vi "RTS Final Station Setups.vi"(0 "Freezer":T4[](array[typedef]) {"Start Time" format="%<%X\n%x>T"; "End Time" format="%<%X\n%x>T"}, 1 "All Door Opener Ctrl in":T1 {"Station 8"."Station Slide"."Chamber 1-1"."Start Time" format="%<%X\n%x>T"; "Station 8"."Station Slide"."Chamber 1-1"."End Time" format="%<%X\n%x>T"; "Station 8"."Station Slide"."Time Count (s)" format="%.2f"; "Station 8"."Station Cab"."Chamber 1-1"."Start Time" format="%<%X\n%x>T"; "Station 8"."Station Cab"."Chamber 1-1"."End Time" format="%<%X\n%x>T"; "Station 8"."Station Cab"."Time Count (s)" format="%.2f"; "Station 8"."Station Freezer"."Chamber 1-1"."Start Time" format="%<%X\n%x>T"; "Station 8"."Station Freezer"."Chamber 1-1"."End Time" format="%<%X\n%x>T"; "Station 8"."Station Freezer"."Time Count (s)" format="%.2f"; "Station 7"."Station Slide"."Chamber 1-1"."Start Time" format="%<%X\n%x>T"; "Station 7"."Station Slide"."Chamber 1-1"."End Time" format="%<%X\n%x>T"; "Station 7"."Station Slide"."Time Count (s)" format="%.2f"; "Station 7"."Station Cab"."Chamber 1-1"."Start Time" format="%<%X\n%x>T"; "Station 7"."Station Cab"."Chamber 1-1"."End Time" format="%<%X\n%x>T"; "Station 7"."Station Cab"."Time Count (s)" format="%.2f"; "Station 7"."Station Freezer"."Chamber 1-1"."Start Time" format="%<%X\n%x>T"; "Station 7"."Station Freezer"."Chamber 1-1"."End Time" format="%<%X\n%x>T"; "Station 7"."Station Freezer"."Time Count (s)" format="%.2f"; "Station 6"."Station Slide"."Chamber 1-1"."Start Time" format="%<%X\n%x>T"; "Station 6"."Station Slide"."Chamber 1-1"."End Time" format="%<%X\n%x>T"; "Station 6"."Station Slide"."Time Count (s)" format="%.2f"; "Station 6"."Station Cab"."Chamber 1-1"."Start Time" format="%<%X\n%x>T"; "Station 6"."Station Cab"."Chamber 1-1"."End Time" format="%<%X\n%x>T"; "Station 6"."Station Cab"."Time Count (s)" format="%.2f"; "Station 6"."Station Freezer"."Chamber 1-1"."Start Time" format="%<%X\n%x>T"; "Station 6"."Station Freezer"."Chamber 1-1"."End Time" format="%<%X\n%x>T"; "Station 6"."Station Freezer"."Time Count (s)" format="%.2f"; "Station 5"."Station Slide"."Chamber 1-1"."Start Time" format="%<%X\n%x>T"; "Station 5"."Station Slide"."Chamber 1-1"."End Time" format="%<%X\n%x>T"; "Station 5"."Station Slide"."Time Count (s)" format="%.2f"; "Station 5"."Station Cab"."Chamber 1-1"."Start Time" format="%<%X\n%x>T"; "Station 5"."Station Cab"."Chamber 1-1"."End Time" format="%<%X\n%x>T"; "Station 5"."Station Cab"."Time Count (s)" format="%.2f"; "Station 5"."Station Freezer"."Chamber 1-1"."Start Time" format="%<%X\n%x>T"; "Station 5"."Station Freezer"."Chamber 1-1"."End Time" format="%<%X\n%x>T"; "Station 5"."Station Freezer"."Time Count (s)" format="%.2f"; "Station 4"."Station Slide"."Chamber 1-1"."Start Time" format="%<%X\n%x>T"; "Station 4"."Station Slide"."Chamber 1-1"."End Time" format="%<%X\n%x>T"; "Station 4"."Station Slide"."Time Count (s)" format="%.2f"; "Station 4"."Station Cab"."Chamber 1-1"."Start Time" format="%<%X\n%x>T"; "Station 4"."Station Cab"."Chamber 1-1"."End Time" format="%<%X\n%x>T"; "Station 4"."Station Cab"."Time Count (s)" format="%.2f"; "Station 4"."Station Freezer"."Chamber 1-1"."Start Time" format="%<%X\n%x>T"; "Station 4"."Station Freezer"."Chamber 1-1"."End Time" format="%<%X\n%x>T"; "Station 4"."Station Freezer"."Time Count (s)" format="%.2f"; "Station 3"."Station Slide"."Chamber 1-1"."Start Time" format="%<%X\n%x>T"; "Station 3"."Station Slide"."Chamber 1-1"."End Time" format="%<%X\n%x>T"; "Station 3"."Station Slide"."Time Count (s)" format="%.2f"; "Station 3"."Station Cab"."Chamber 1-1"."Start Time" format="%<%X\n%x>T"; "Station 3"."Station Cab"."Chamber 1-1"."End Time" format="%<%X\n%x>T"; "Station 3"."Station Cab"."Time Count (s)" format="%.2f"; "Station 3"."Station Freezer"."Chamber 1-1"."Start Time" format="%<%X\n%x>T"; "Station 3"."Station Freezer"."Chamber 1-1"."End Time" format="%<%X\n%x>T"; "Station 3"."Station Freezer"."Time Count (s)" format="%.2f"; "Station 2"."Station Slide"."Chamber 1-1"."Start Time" format="%<%X\n%x>T"; "Station 2"."Station Slide"."Chamber 1-1"."End Time" format="%<%X\n%x>T"; "Station 2"."Station Slide"."Time Count (s)" format="%.2f"; "Station 2"."Station Cab"."Chamber 1-1"."Start Time" format="%<%X\n%x>T"; "Station 2"."Station Cab"."Chamber 1-1"."End Time" format="%<%X\n%x>T"; "Station 2"."Station Cab"."Time Count (s)" format="%.2f"; "Station 2"."Station Freezer"."Chamber 1-1"."Start Time" format="%<%X\n%x>T"; "Station 2"."Station Freezer"."Chamber 1-1"."End Time" format="%<%X\n%x>T"; "Station 2"."Station Freezer"."Time Count (s)" format="%.2f"; "Station 1"."Station Slide"."Chamber 1-1"."Start Time" format="%<%X\n%x>T"; "Station 1"."Station Slide"."Chamber 1-1"."End Time" format="%<%X\n%x>T"; "Station 1"."Station Slide"."Time Count (s)" format="%.2f"; "Station 1"."Station Cab"."Chamber 1-1"."Start Time" format="%<%X\n%x>T"; "Station 1"."Station Cab"."Chamber 1-1"."End Time" format="%<%X\n%x>T"; "Station 1"."Station Cab"."Time Count (s)" format="%.2f"; "Station 1"."Station Freezer"."Chamber 1-1"."Start Time" format="%<%X\n%x>T"; "Station 1"."Station Freezer"."Chamber 1-1"."End Time" format="%<%X\n%x>T"; "Station 1"."Station Freezer"."Time Count (s)" format="%.2f"}, 2 "Station #":u8, 5 "Cab":T4[](array[typedef]) {"Start Time" format="%<%X\n%x>T"; "End Time" format="%<%X\n%x>T"}, 7 "Slide":T4[](array[typedef]) {"Start Time" format="%<%X\n%x>T"; "End Time" format="%<%X\n%x>T"}, 9 "RTS Config Setup Input":T7, 11 "Error In":errorcluster, 12 "Slide Index":i32, 13 "Cab Index":i32, 14 "Freezer Index":i32) -> (3 "All Door Opener Ctrl Out":T1={"Station 1"={"Station Freezer"={"Time Count (s)"=0.0, "Status"="", "Door State"=FALSE, "Delay"=FALSE, "Chamber 1-1"=[], "Index"=0, "Delay Status"=""}, "Station Cab"={"Time Count (s)"=0.0, "Status"="", "Door State"=FALSE, "Delay"=FALSE, "Chamber 1-1"=[], "Index"=0, "Delay Status"=""}, "Station Slide"={"Time Count (s)"=0.0, "Status"="", "Door State"=FALSE, "Delay"=FALSE, "Chamber 1-1"=[], "Index"=0, "Delay Status"=""}, "1st Complete"=FALSE, "2nd Complete"=FALSE, "3rd Complete"=FALSE}, "Station 2"={"Station Freezer"={"Time Count (s)"=0.0, "Status"="", "Door State"=FALSE, "Delay"=FALSE, "Chamber 1-1"=[], "Index"=0, "Delay Status"=""}, "Station Cab"={"Time Count (s)"=0.0, "Status"="", "Door State"=FALSE, "Delay"=FALSE, "Chamber 1-1"=[], "Index"=0, "Delay Status"=""}, "Station Slide"={"Time Count (s)"=0.0, "Status"="", "Door State"=FALSE, "Delay"=FALSE, "Chamber 1-1"=[], "Index"=0, "Delay Status"=""}, "1st Complete"=FALSE, "2nd Complete"=FALSE, "3rd Complete"=FALSE}, "Station 3"={"Station Freezer"={"Time Count (s)"=0.0, "Status"="", "Door State"=FALSE, "Delay"=FALSE, "Chamber 1-1"=[], "Index"=0, "Delay Status"=""}, "Station Cab"={"Time Count (s)"=0.0, "Status"="", "Door State"=FALSE, "Delay"=FALSE, "Chamber 1-1"=[], "Index"=0, "Delay Status"=""}, "Station Slide"={"Time Count (s)"=0.0, "Status"="", "Door State"=FALSE, "Delay"=FALSE, "Chamber 1-1"=[], "Index"=0, "Delay Status"=""}, "1st Complete"=FALSE, "2nd Complete"=FALSE, "3rd Complete"=FALSE}, "Station 4"={"Station Freezer"={"Time Count (s)"=0.0, "Status"="", "Door State"=FALSE, "Delay"=FALSE, "Chamber 1-1"=[], "Index"=0, "Delay Status"=""}, "Station Cab"={"Time Count (s)"=0.0, "Status"="", "Door State"=FALSE, "Delay"=FALSE, "Chamber 1-1"=[], "Index"=0, "Delay Status"=""}, "Station Slide"={"Time Count (s)"=0.0, "Status"="", "Door State"=FALSE, "Delay"=FALSE, "Chamber 1-1"=[], "Index"=0, "Delay Status"=""}, "1st Complete"=FALSE, "2nd Complete"=FALSE, "3rd Complete"=FALSE}, "Station 5"={"Station Freezer"={"Time Count (s)"=0.0, "Status"="", "Door State"=FALSE, "Delay"=TRUE, "Chamber 1-1"=[], "Index"=0, "Delay Status"=""}, "Station Cab"={"Time Count (s)"=0.0, "Status"="", "Door State"=FALSE, "Delay"=TRUE, "Chamber 1-1"=[], "Index"=0, "Delay Status"=""}, "Station Slide"={"Time Count (s)"=0.0, "Status"="", "Door State"=FALSE, "Delay"=TRUE, "Chamber 1-1"=[], "Index"=0, "Delay Status"=""}, "1st Complete"=FALSE, "2nd Complete"=FALSE, "3rd Complete"=FALSE}, "Station 6"={"Station Freezer"={"Time Count (s)"=0.0, "Status"="", "Door State"=FALSE, "Delay"=TRUE, "Chamber 1-1"=[], "Index"=0, "Delay Status"=""}, "Station Cab"={"Time Count (s)"=0.0, "Status"="", "Door State"=FALSE, "Delay"=TRUE, "Chamber 1-1"=[], "Index"=0, "Delay Status"=""}, "Station Slide"={"Time Count (s)"=0.0, "Status"="", "Door State"=FALSE, "Delay"=TRUE, "Chamber 1-1"=[], "Index"=0, "Delay Status"=""}, "1st Complete"=FALSE, "2nd Complete"=FALSE, "3rd Complete"=FALSE}, "Station 7"={"Station Freezer"={"Time Count (s)"=0.0, "Status"="", "Door State"=FALSE, "Delay"=TRUE, "Chamber 1-1"=[], "Index"=0, "Delay Status"=""}, "Station Cab"={"Time Count (s)"=0.0, "Status"="", "Door State"=FALSE, "Delay"=TRUE, "Chamber 1-1"=[], "Index"=0, "Delay Status"=""}, "Station Slide"={"Time Count (s)"=0.0, "Status"="", "Door State"=FALSE, "Delay"=TRUE, "Chamber 1-1"=[], "Index"=0, "Delay Status"=""}, "1st Complete"=FALSE, "2nd Complete"=FALSE, "3rd Complete"=FALSE}, "Station 8"={"Station Freezer"={"Time Count (s)"=0.0, "Status"="", "Door State"=FALSE, "Delay"=TRUE, "Chamber 1-1"=[], "Index"=0, "Delay Status"=""}, "Station Cab"={"Time Count (s)"=0.0, "Status"="", "Door State"=FALSE, "Delay"=TRUE, "Chamber 1-1"=[], "Index"=0, "Delay Status"=""}, "Station Slide"={"Time Count (s)"=0.0, "Status"="", "Door State"=FALSE, "Delay"=TRUE, "Chamber 1-1"=[], "Index"=0, "Delay Status"=""}, "1st Complete"=FALSE, "2nd Complete"=FALSE, "3rd Complete"=FALSE}} {"Station 8"."Station Slide"."Chamber 1-1"."Start Time" format="%<%X\n%x>T"; "Station 8"."Station Slide"."Chamber 1-1"."End Time" format="%<%X\n%x>T"; "Station 8"."Station Slide"."Time Count (s)" format="%.2f"; "Station 8"."Station Cab"."Chamber 1-1"."Start Time" format="%<%X\n%x>T"; "Station 8"."Station Cab"."Chamber 1-1"."End Time" format="%<%X\n%x>T"; "Station 8"."Station Cab"."Time Count (s)" format="%.2f"; "Station 8"."Station Freezer"."Chamber 1-1"."Start Time" format="%<%X\n%x>T"; "Station 8"."Station Freezer"."Chamber 1-1"."End Time" format="%<%X\n%x>T"; "Station 8"."Station Freezer"."Time Count (s)" format="%.2f"; "Station 7"."Station Slide"."Chamber 1-1"."Start Time" format="%<%X\n%x>T"; "Station 7"."Station Slide"."Chamber 1-1"."End Time" format="%<%X\n%x>T"; "Station 7"."Station Slide"."Time Count (s)" format="%.2f"; "Station 7"."Station Cab"."Chamber 1-1"."Start Time" format="%<%X\n%x>T"; "Station 7"."Station Cab"."Chamber 1-1"."End Time" format="%<%X\n%x>T"; "Station 7"."Station Cab"."Time Count (s)" format="%.2f"; "Station 7"."Station Freezer"."Chamber 1-1"."Start Time" format="%<%X\n%x>T"; "Station 7"."Station Freezer"."Chamber 1-1"."End Time" format="%<%X\n%x>T"; "Station 7"."Station Freezer"."Time Count (s)" format="%.2f"; "Station 6"."Station Slide"."Chamber 1-1"."Start Time" format="%<%X\n%x>T"; "Station 6"."Station Slide"."Chamber 1-1"."End Time" format="%<%X\n%x>T"; "Station 6"."Station Slide"."Time Count (s)" format="%.2f"; "Station 6"."Station Cab"."Chamber 1-1"."Start Time" format="%<%X\n%x>T"; "Station 6"."Station Cab"."Chamber 1-1"."End Time" format="%<%X\n%x>T"; "Station 6"."Station Cab"."Time Count (s)" format="%.2f"; "Station 6"."Station Freezer"."Chamber 1-1"."Start Time" format="%<%X\n%x>T"; "Station 6"."Station Freezer"."Chamber 1-1"."End Time" format="%<%X\n%x>T"; "Station 6"."Station Freezer"."Time Count (s)" format="%.2f"; "Station 5"."Station Slide"."Chamber 1-1"."Start Time" format="%<%X\n%x>T"; "Station 5"."Station Slide"."Chamber 1-1"."End Time" format="%<%X\n%x>T"; "Station 5"."Station Slide"."Time Count (s)" format="%.2f"; "Station 5"."Station Cab"."Chamber 1-1"."Start Time" format="%<%X\n%x>T"; "Station 5"."Station Cab"."Chamber 1-1"."End Time" format="%<%X\n%x>T"; "Station 5"."Station Cab"."Time Count (s)" format="%.2f"; "Station 5"."Station Freezer"."Chamber 1-1"."Start Time" format="%<%X\n%x>T"; "Station 5"."Station Freezer"."Chamber 1-1"."End Time" format="%<%X\n%x>T"; "Station 5"."Station Freezer"."Time Count (s)" format="%.2f"; "Station 4"."Station Slide"."Chamber 1-1"."Start Time" format="%<%X\n%x>T"; "Station 4"."Station Slide"."Chamber 1-1"."End Time" format="%<%X\n%x>T"; "Station 4"."Station Slide"."Time Count (s)" format="%.2f"; "Station 4"."Station Cab"."Chamber 1-1"."Start Time" format="%<%X\n%x>T"; "Station 4"."Station Cab"."Chamber 1-1"."End Time" format="%<%X\n%x>T"; "Station 4"."Station Cab"."Time Count (s)" format="%.2f"; "Station 4"."Station Freezer"."Chamber 1-1"."Start Time" format="%<%X\n%x>T"; "Station 4"."Station Freezer"."Chamber 1-1"."End Time" format="%<%X\n%x>T"; "Station 4"."Station Freezer"."Time Count (s)" format="%.2f"; "Station 3"."Station Slide"."Chamber 1-1"."Start Time" format="%<%X\n%x>T"; "Station 3"."Station Slide"."Chamber 1-1"."End Time" format="%<%X\n%x>T"; "Station 3"."Station Slide"."Time Count (s)" format="%.2f"; "Station 3"."Station Cab"."Chamber 1-1"."Start Time" format="%<%X\n%x>T"; "Station 3"."Station Cab"."Chamber 1-1"."End Time" format="%<%X\n%x>T"; "Station 3"."Station Cab"."Time Count (s)" format="%.2f"; "Station 3"."Station Freezer"."Chamber 1-1"."Start Time" format="%<%X\n%x>T"; "Station 3"."Station Freezer"."Chamber 1-1"."End Time" format="%<%X\n%x>T"; "Station 3"."Station Freezer"."Time Count (s)" format="%.2f"; "Station 2"."Station Slide"."Chamber 1-1"."Start Time" format="%<%X\n%x>T"; "Station 2"."Station Slide"."Chamber 1-1"."End Time" format="%<%X\n%x>T"; "Station 2"."Station Slide"."Time Count (s)" format="%.2f"; "Station 2"."Station Cab"."Chamber 1-1"."Start Time" format="%<%X\n%x>T"; "Station 2"."Station Cab"."Chamber 1-1"."End Time" format="%<%X\n%x>T"; "Station 2"."Station Cab"."Time Count (s)" format="%.2f"; "Station 2"."Station Freezer"."Chamber 1-1"."Start Time" format="%<%X\n%x>T"; "Station 2"."Station Freezer"."Chamber 1-1"."End Time" format="%<%X\n%x>T"; "Station 2"."Station Freezer"."Time Count (s)" format="%.2f"; "Station 1"."Station Slide"."Chamber 1-1"."Start Time" format="%<%X\n%x>T"; "Station 1"."Station Slide"."Chamber 1-1"."End Time" format="%<%X\n%x>T"; "Station 1"."Station Slide"."Time Count (s)" format="%.2f"; "Station 1"."Station Cab"."Chamber 1-1"."Start Time" format="%<%X\n%x>T"; "Station 1"."Station Cab"."Chamber 1-1"."End Time" format="%<%X\n%x>T"; "Station 1"."Station Cab"."Time Count (s)" format="%.2f"; "Station 1"."Station Freezer"."Chamber 1-1"."Start Time" format="%<%X\n%x>T"; "Station 1"."Station Freezer"."Chamber 1-1"."End Time" format="%<%X\n%x>T"; "Station 1"."Station Freezer"."Time Count (s)" format="%.2f"}, 4 "States":string, 10 "RTS Config Setup Output":T7, 15 "Error Out":errorcluster)   [LabVIEW 2016]
uses:
  Type Definitions/RTS All Station Door Opener Ctrl.ctl
  Type Definitions/RTS Station Relay Ops.ctl
  Type Definitions/RTS Door Opener Indicator.ctl
  Type Definitions/RTS Door Ops Client.ctl
  Type Definitions/RTS Door Opening Schedule.ctl
  Type Definitions/RTS Door Ops Sequence.ctl
  Type Definitions/RTS Configuration Setup.ctl
  Type Definitions/RTS Wago Config.ctl
  Type Definitions/RTS APLUS Config.ctl
  Type Definitions/RTS Yokogawa MX Config.ctl
  Type Definitions/RTS Replay Server Control.ctl
  Type Definitions/RTS Server Configuration.ctl
  Type Definitions/RTS Station Settions TCP Comms.ctl
  Type Definitions/RTS Chamber Save Status.ctl
  Type Definitions/RTS Test Pattern.ctl
panel:
  # "Chamber Conditions:"
  # "Chamber Conditions:"
  # "Chamber Conditions:"
  # "Chamber Conditions:"
  # "Chamber Conditions:"
  # "Chamber Conditions:"
  # "Chamber Conditions:"
  # "Chamber Conditions:"
  # "Chamber Conditions:"
  # "Chamber Conditions:"
  # "Chamber Conditions:"
  # "Chamber Conditions:"
  # "Chamber Conditions:"
  # "Chamber Conditions:"
  # "Chamber Conditions:"
  # "Chamber Conditions:"
  # "Chamber Conditions:"
  # "Chamber Conditions:"
  # "Chamber Conditions:"
  # "Chamber Conditions:"
  # "Chamber Conditions:"
  # "Chamber Conditions:"
  # "Chamber Conditions:"
  # "Chamber Conditions:"
  # "Chamber Conditions:"
  # "Chamber Conditions:"
  # "Chamber Conditions:"
  # "Chamber Conditions:"
  # "Chamber Conditions:"
  # "Chamber Conditions:"
  # "Chamber Conditions:"
  # "Chamber Conditions:"
  # "Chamber Conditions:"
  # "Chamber Conditions:"
  # "Chamber Conditions:"
  # "Chamber Conditions:"
  # "Chamber Conditions:"
  # "Chamber Conditions:"
  # "Chamber Conditions:"
  # "Chamber Conditions:"
  # "Chamber Conditions:"
  # "Chamber Conditions:"
  # "Chamber Conditions:"
  # "Chamber Conditions:"
  # "Chamber Conditions:"
  # "Chamber Conditions:"
  # "Chamber Conditions:"
  # "Chamber Conditions:"
  # "Chamber Conditions:"
  # "Chamber Conditions:"
  # "Chamber Conditions:"
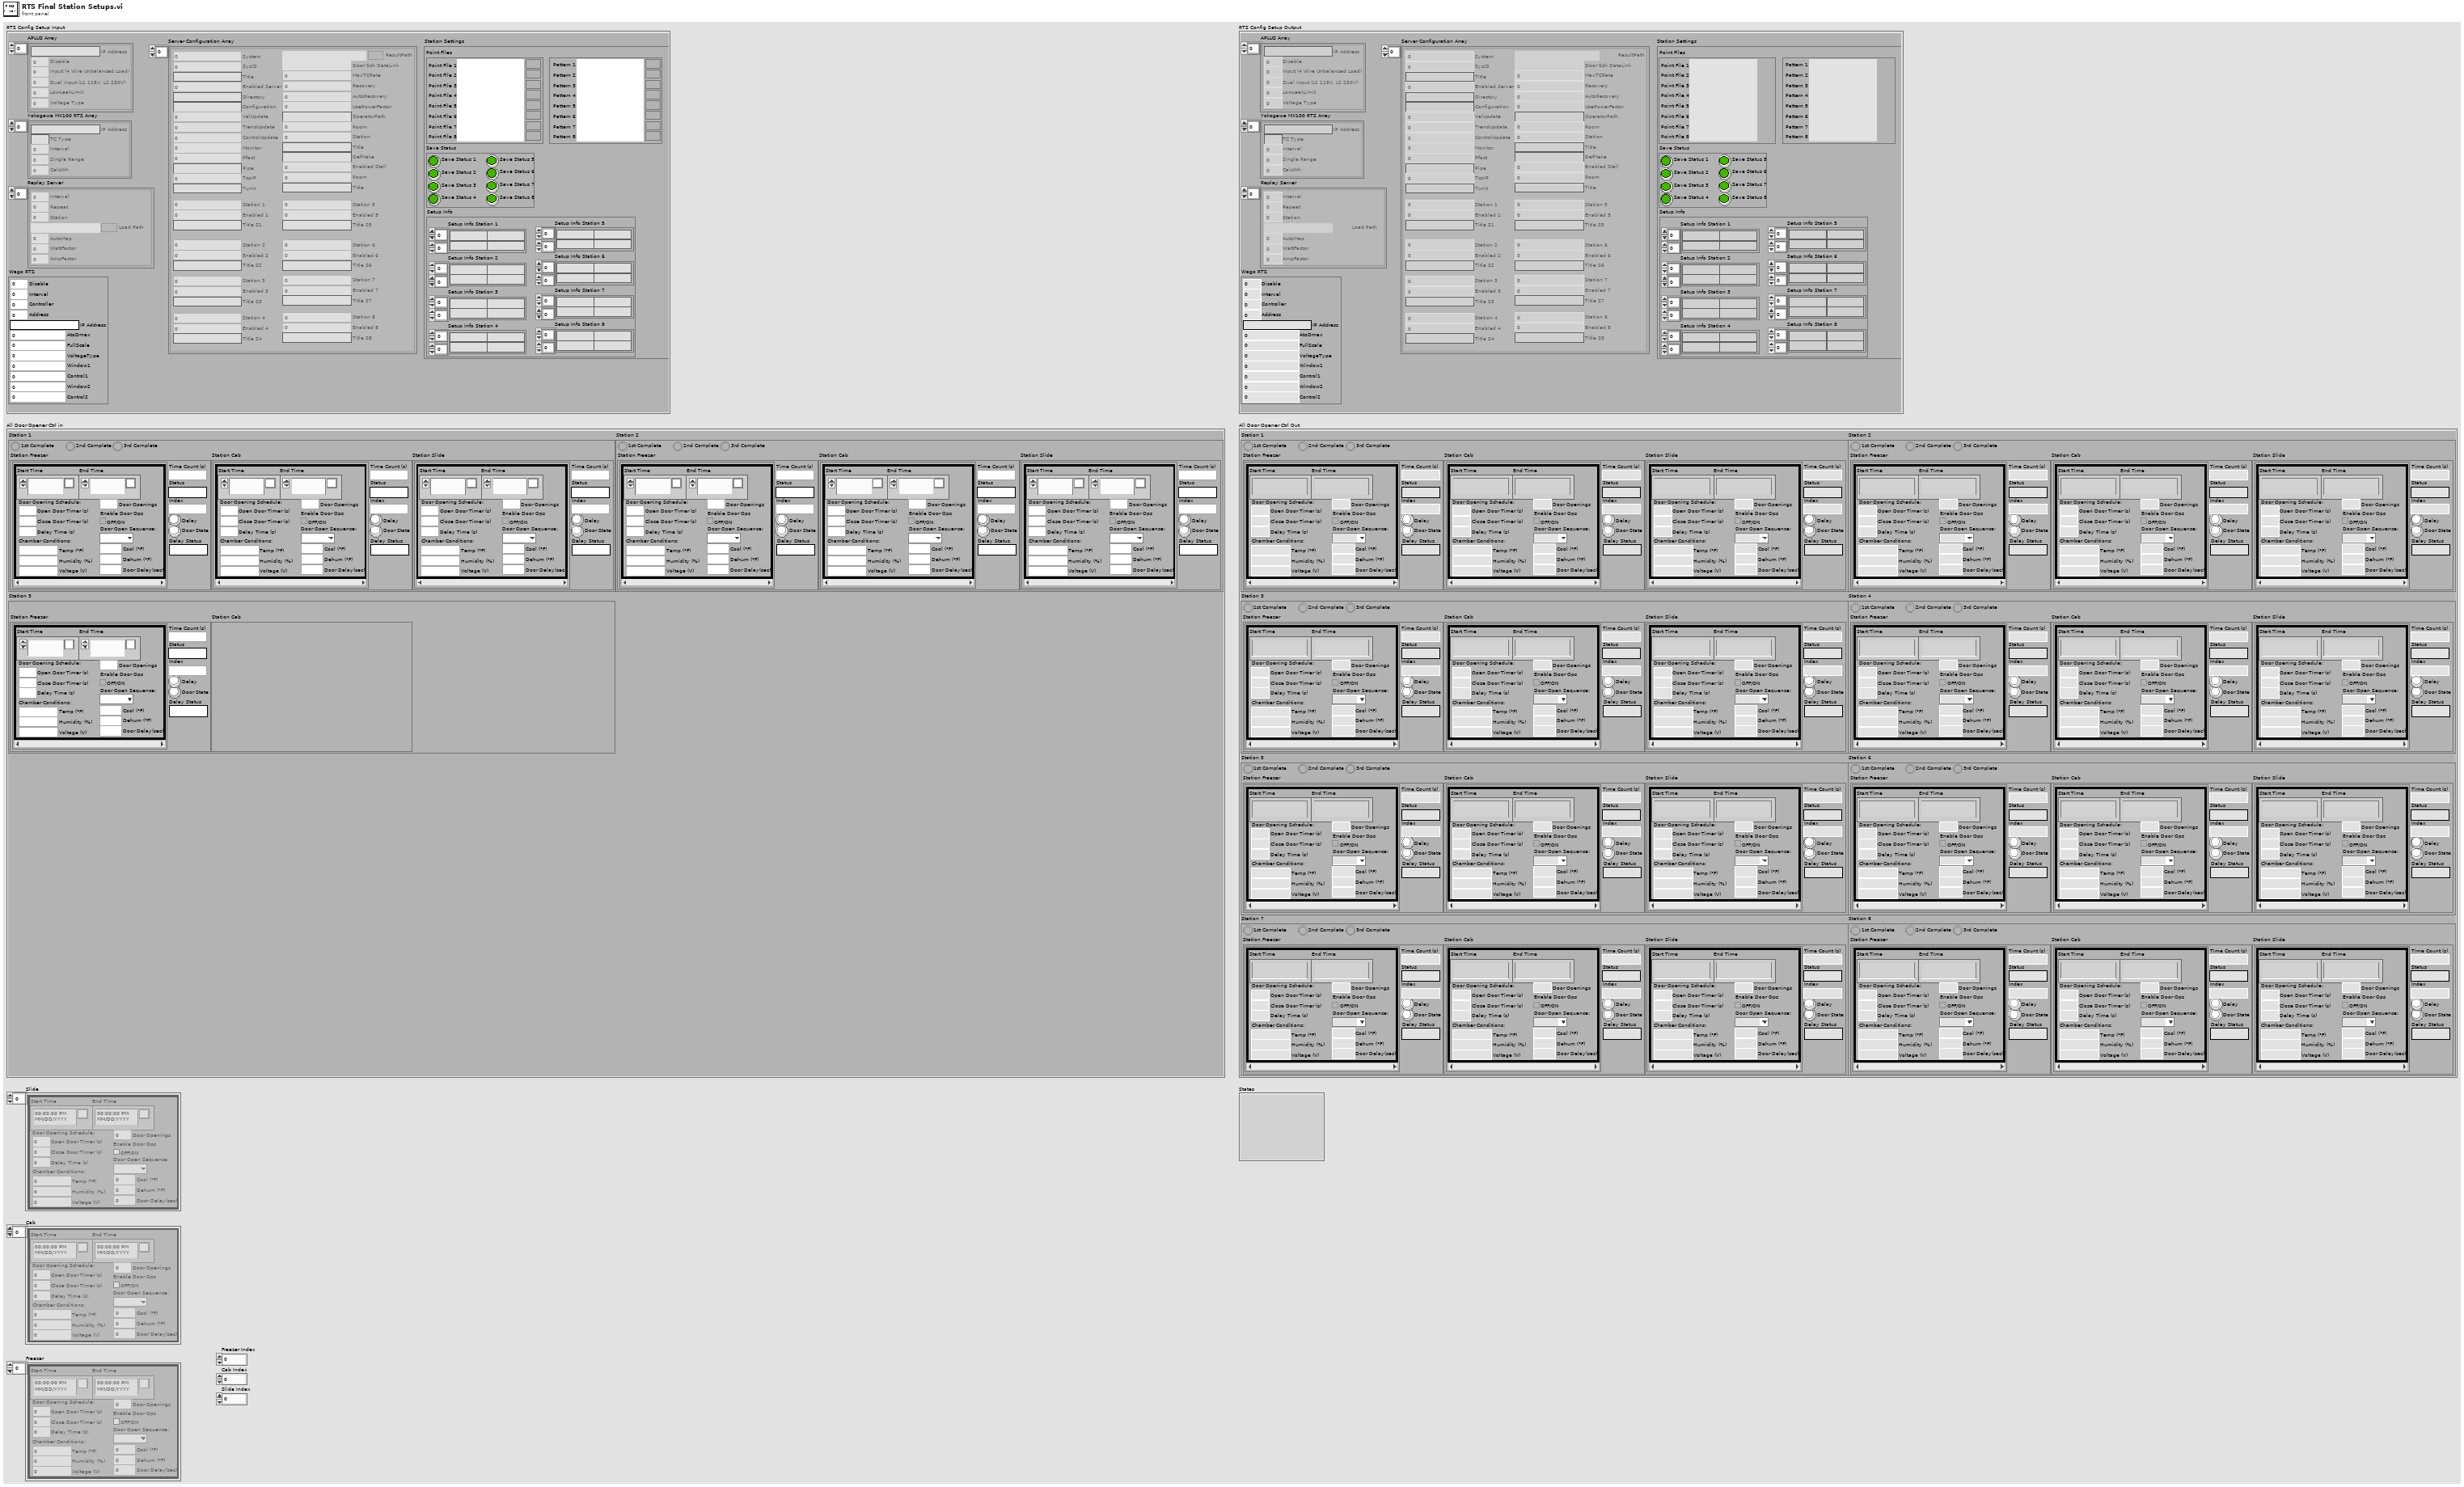
[diagram p1: front panel]
types:
  T1 = typedef "RTS All Station Door Opener Ctrl.ctl" = cluster{"Station 1":T2, "Station 2":T2, "Station 3":T2, "Station 4":T2, "Station 5":T2, "Station 6":T2, "Station 7":T2, "Station 8":T2}
  T2 = typedef "RTS Station Relay Ops.ctl" = cluster{"Station Freezer":T3, "Station Cab":T3, "Station Slide":T3, "1st Complete":bool, "2nd Complete":bool, "3rd Complete":bool}
  T3 = typedef "RTS Door Opener Indicator.ctl" = cluster{"Time Count (s)":dbl, "Status":string, "Door State":bool, "Delay":bool, "Chamber 1-1":T4[], "Index":i32, "Delay Status":string}
  T4 = typedef "RTS Door Ops Client.ctl" = cluster{"End Time":timestamp, "Start Time":timestamp, "Door Opening Schedule:":T5, "Enable Door Ops":bool, "Door Openings":u32, "Temp (°F)":dbl, "Humidity (%)":dbl, "Voltage (V)":dbl, "Door Open Sequence:":T6, "Door Delay(sec)":dbl, "Dehum (°F)":dbl, "Cool (°F)":dbl}
  T5 = typedef "RTS Door Opening Schedule.ctl" = cluster{"Open Door Timer (s)":dbl, "Delay Time (s)":dbl, "Close Door Timer (s)":dbl}
  T6 = typedef "RTS Door Ops Sequence.ctl" = enum16{"", "1st", "2nd", "3rd"}
  T7 = typedef "RTS Configuration Setup.ctl" = cluster{"Wago RTS":T8, "APLUS Array":T9[], "Yokogawa MX100 RTS Array":T10[], "Replay Server":T11[], "Server Configuration Array":T12[], "Station Settings":T13}
  T8 = typedef "RTS Wago Config.ctl" = cluster{"Disable":u16, "Interval":u16, "Controller":u16, "Address":u16, "IP Address":string, "AtoDmax":u16, "FullScale":u16, "VoltageType":u16, "Window1":u16, "Control1":u16, "Window2":u16, "Control2":u16}
  T9 = typedef "RTS APLUS Config.ctl" = cluster{"Disable":u16, "IP Address":string, "Input (4 Wire Unbalanced Load)":u16, "Dual Input (L1 115V, L2 230V)":u16, "LowLeakLimit":dbl, "Voltage Type":u16}
  T10 = typedef "RTS Yokogawa MX Config.ctl" = cluster{"IP Address":string, "TC Type":string, "Interval":u16, "Single Range":u16, "CalcWh":u16}
  T11 = typedef "RTS Replay Server Control.ctl" = cluster{"Interval":i16, "Repeat":u16, "Station":u16, "Load Path":path, "AutoMap":u16, "WattFactor":dbl, "AmpFactor":dbl}
  T12 = typedef "RTS Server Configuration.ctl" = cluster{"System":u16, "SysID":u16, "Title":string, "Enabled Server":u16, "Directory":string, "Configuration":string, "ValUpdate":u16, "TrendUpdate":u16, "ControlUpdate":u16, "Monitor":u16, "Pfact":u16, "Pipe":string, "TcpIP":u16, "Tunit":string, "ResultPath":path, "Door Sch DataLink":path, "MaxTCRate":u16, "Recovery":u16, "AutoRecovery":u16, "UsePowerFactor":u16, "OperatorPath":string, "Room":u16, "Station":u16, "Title":string, "DefMake":string, "Enabled Stall":u16, "Room":u16, "Title":string, "Station 1":u16, "Enabled 1":u16, "Station 2":u16, "Enabled 2":u16, "Station 3":u16, "Enabled 3":u16, "Station 4":u16, "Enabled 4":u16, "Station 5":u16, "Enabled 5":u16, "Station 6":u16, "Enabled 6":u16, "Station 7":u16, "Enabled 7":u16, "Station 8":u16, "Enabled 8":u16, "Title S1":string, "Title S2":string, "Title S3":string, "Title S5":string, "Title S6":string, "Title S7":string, "Title S8":string, "Title S4":string}
  T13 = typedef "RTS Station Settions TCP Comms.ctl" = cluster{"Point Files":cluster{"Point File 1":path, "Point File 2":path, "Point File 3":path, "Point File 4":path, "Point File 5":path, "Point File 6":path, "Point File 7":path, "Point File 8":path}, "Save Status":T14, "Setup Info":cluster{"Setup Info Station 1":string[][], "Setup Info Station 2":string[][], "Setup Info Station 3":string[][], "Setup Info Station 4":string[][], "Setup Info Station 5":string[][], "Setup Info Station 6":string[][], "Setup Info Station 7":string[][], "Setup Info Station 8":string[][]}, "Chamber Test Pattern":T15}
  T14 = typedef "RTS Chamber Save Status.ctl" = cluster{"Save Status 1":bool, "Save Status 2":bool, "Save Status 3":bool, "Save Status 4":bool, "Save Status 5":bool, "Save Status 6":bool, "Save Status 7":bool, "Save Status 8":bool}
  T15 = typedef "RTS Test Pattern.ctl" = cluster{" Pattern 1":path, "Pattern 2":path, "Pattern 3":path, "Pattern 4":path, "Pattern 5":path, "Pattern 6":path, "Pattern 7":path, "Pattern 8":path}
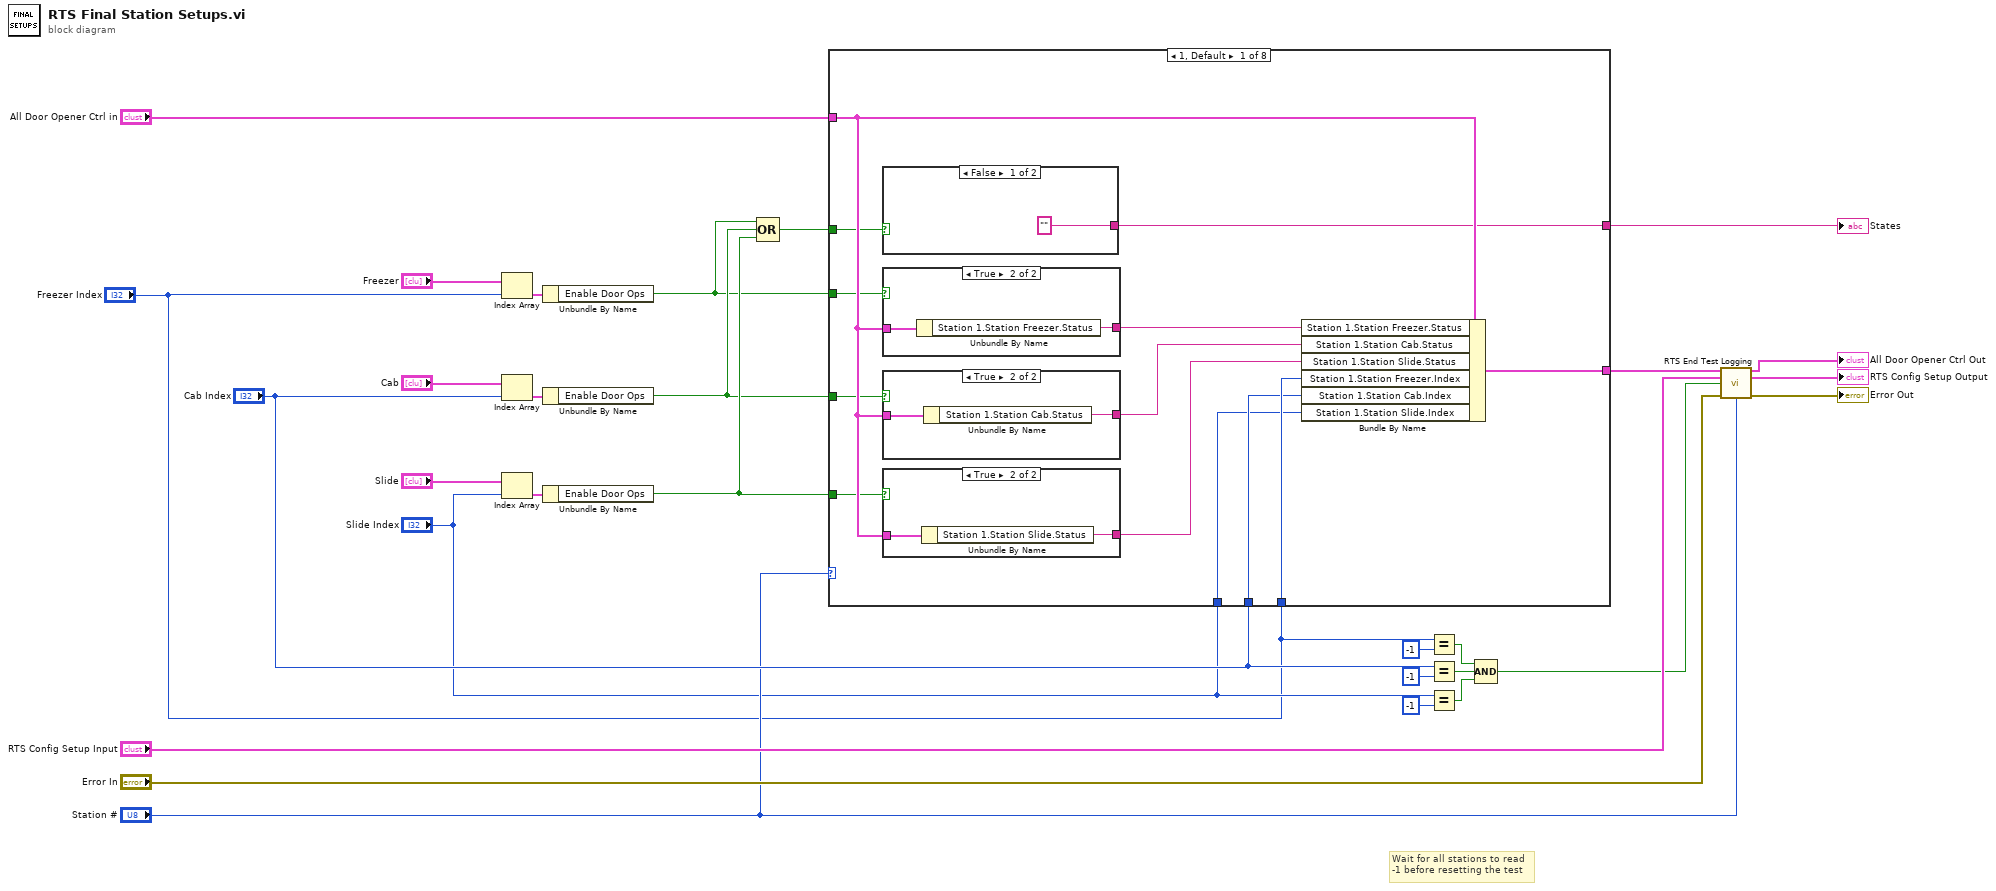
[diagram p0: block diagram]
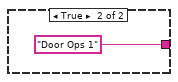
[diagram p2: hidden frame]
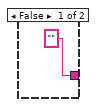
[diagram p3: hidden frame]
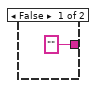
[diagram p4: hidden frame]
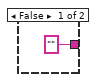
[diagram p5: hidden frame]
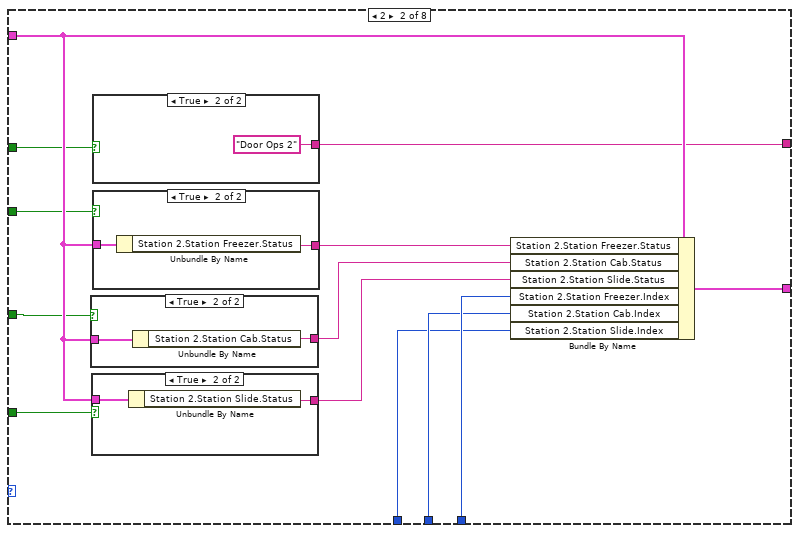
[diagram p6: hidden frame]
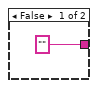
[diagram p7: hidden frame]
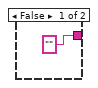
[diagram p8: hidden frame]
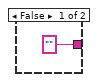
[diagram p9: hidden frame]
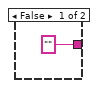
[diagram p10: hidden frame]
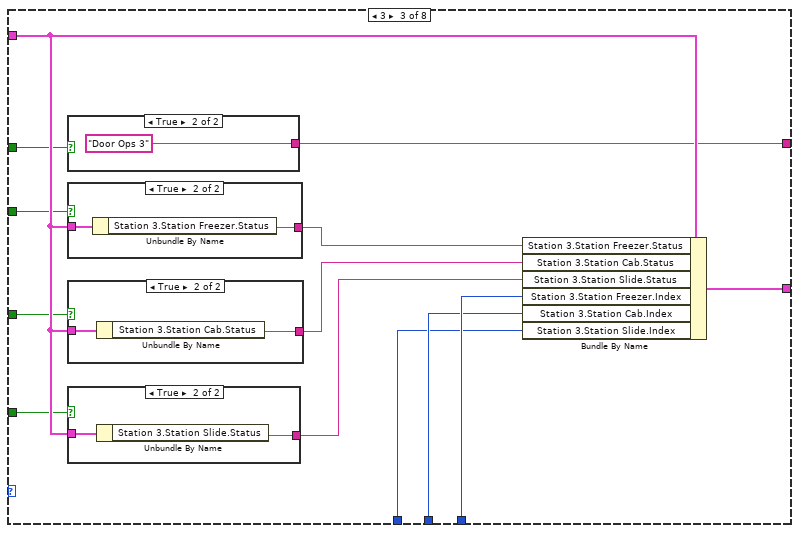
[diagram p11: hidden frame]
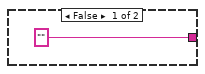
[diagram p12: hidden frame]
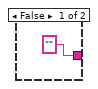
[diagram p13: hidden frame]
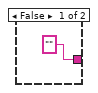
[diagram p14: hidden frame]
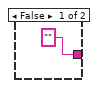
[diagram p15: hidden frame]
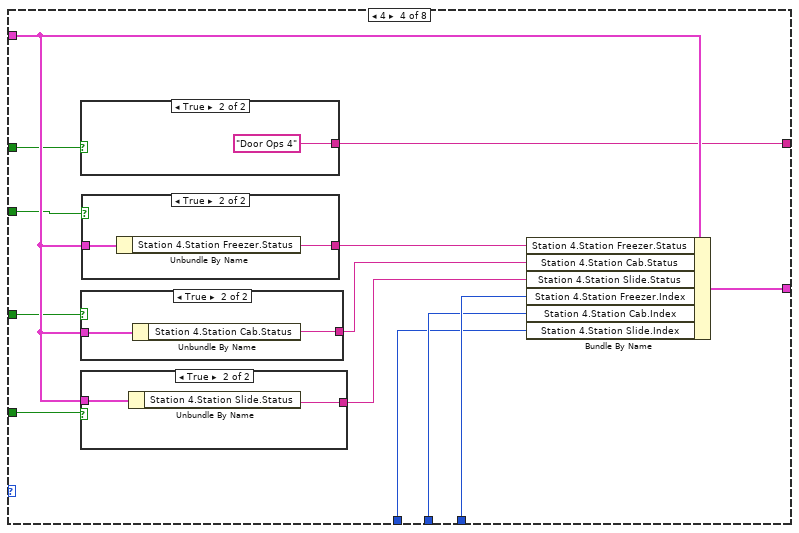
[diagram p16: hidden frame]
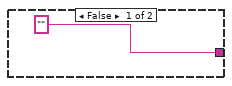
[diagram p17: hidden frame]
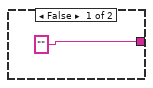
[diagram p18: hidden frame]
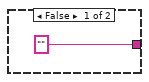
[diagram p19: hidden frame]
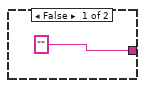
[diagram p20: hidden frame]
diagram:
  # "Wait for all stations to read\n-1 before resetting the test"
  n1 = Index Array(array="Freezer", index="Freezer Index") -> (element=w19:T4)
  n2 = Index Array(array="Cab", index="Cab Index") -> (element=w21:T4)
  n3 = Index Array(array="Slide", index="Slide Index") -> (element=w20:T4)
  n4 = Unbundle By Name(w19) -> ("Enable Door Ops"=w22:bool)
  n5 = Unbundle By Name(w21) -> ("Enable Door Ops"=w23:bool)
  n6 = Unbundle By Name(w20) -> ("Enable Door Ops"=w24:bool)
  n7 = Compound Arithmetic op=OR(w22, w23, w24) -> (w17:bool)
  n8 = case shown="1, Default" "Station #" {
    tunnel: "All Door Opener Ctrl in" -> [w39 w63 w87 w110 w134 w158 w183 w207]
    tunnel: w24 -> [w38 w55 w86 w106 w133 w157 w179 w203]
    tunnel: w23 -> [w37 w56 w85 w107 w132 w156 w178 w202]
    tunnel: w22 -> [w36 w57 w84 w108 w131 w155 w177 w201]
    tunnel: [w35 w62 w81 w105 w129 w154 w180 w205] -> w18
    tunnel: w17 -> [w34 w54 w83 w109 w130 w153 w181 w204]
    tunnel: "Freezer Index" -> [w33 w60 w80 w104 w128 w152 w176 w200]
    tunnel: "Cab Index" -> [w32 w59 w79 w103 w127 w151 w175 w199]
    tunnel: "Slide Index" -> [w31 w58 w78 w102 w126 w150 w174 w198]
    tunnel: [w30 w61 w82 w111 w135 w159 w182 w206] -> w5
    frame 1, Default {
      n9 = case shown="False" w34 {
        tunnel: ["" ("State(s) in Front (\"\")") "Door Ops 1" ("State(s) in Front (\"\")")] -> w35
        frame False {
        }
        frame True {
        }
      }
      n10 = case shown="True" w36 {
        tunnel: ["" w52] -> w40
        tunnel: w39 -> [_ w53]
        frame False {
        }
        frame True {
          n11 = Unbundle By Name(w53) -> ("Station 1.Station Freezer.Status"=w52:string)
        }
      }
      n12 = case shown="True" w37 {
        tunnel: ["" w49] -> w41
        tunnel: w39 -> [_ w50]
        frame False {
        }
        frame True {
          n13 = Unbundle By Name(w50) -> ("Station 1.Station Cab.Status"=w49:string)
        }
      }
      n14 = case shown="True" w38 {
        tunnel: ["" w46] -> w42
        tunnel: w39 -> [_ w47]
        frame False {
        }
        frame True {
          n15 = Unbundle By Name(w47) -> ("Station 1.Station Slide.Status"=w46:string)
        }
      }
      n16 = Bundle By Name(cluster=w39, "Station 1.Station Freezer.Status"=w40, "Station 1.Station Cab.Status"=w41, "Station 1.Station Slide.Status"=w42, "Station 1.Station Freezer.Index"=w33, "Station 1.Station Cab.Index"=w32, "Station 1.Station Slide.Index"=w31) -> (w30:T1)
    }
    frame 2 {
      n17 = case shown="True" w56 {
        tunnel: ["" w73] -> w65
        tunnel: w63 -> [_ w74]
        frame False {
        }
        frame True {
          n18 = Unbundle By Name(w74) -> ("Station 2.Station Cab.Status"=w73:string)
        }
      }
      n19 = case shown="True" w55 {
        tunnel: ["" w70] -> w66
        tunnel: w63 -> [_ w71]
        frame False {
        }
        frame True {
          n20 = Unbundle By Name(w71) -> ("Station 2.Station Slide.Status"=w70:string)
        }
      }
      n21 = case shown="True" w54 {
        tunnel: ["" ("State(s) in Front (\"\")") "Door Ops 2" ("State(s) in Front (\"\")")] -> w62
        frame False {
        }
        frame True {
        }
      }
      n22 = case shown="True" w57 {
        tunnel: ["" w76] -> w64
        tunnel: w63 -> [_ w77]
        frame False {
        }
        frame True {
          n23 = Unbundle By Name(w77) -> ("Station 2.Station Freezer.Status"=w76:string)
        }
      }
      n24 = Bundle By Name(cluster=w63, "Station 2.Station Freezer.Status"=w64, "Station 2.Station Cab.Status"=w65, "Station 2.Station Slide.Status"=w66, "Station 2.Station Freezer.Index"=w60, "Station 2.Station Cab.Index"=w59, "Station 2.Station Slide.Index"=w58) -> (w61:T1)
    }
    frame 3 {
      n25 = case shown="True" w83 {
        tunnel: ["" ("State(s) in Front (\"\")") "Door Ops 3" ("State(s) in Front (\"\")")] -> w81
        frame False {
        }
        frame True {
        }
      }
      n26 = case shown="True" w84 {
        tunnel: ["" w100] -> w88
        tunnel: w87 -> [_ w101]
        frame False {
        }
        frame True {
          n27 = Unbundle By Name(w101) -> ("Station 3.Station Freezer.Status"=w100:string)
        }
      }
      n28 = case shown="True" w85 {
        tunnel: ["" w97] -> w89
        tunnel: w87 -> [_ w98]
        frame False {
        }
        frame True {
          n29 = Unbundle By Name(w98) -> ("Station 3.Station Cab.Status"=w97:string)
        }
      }
      n30 = case shown="True" w86 {
        tunnel: ["" w94] -> w90
        tunnel: w87 -> [_ w95]
        frame False {
        }
        frame True {
          n31 = Unbundle By Name(w95) -> ("Station 3.Station Slide.Status"=w94:string)
        }
      }
      n32 = Bundle By Name(cluster=w87, "Station 3.Station Freezer.Status"=w88, "Station 3.Station Cab.Status"=w89, "Station 3.Station Slide.Status"=w90, "Station 3.Station Freezer.Index"=w80, "Station 3.Station Cab.Index"=w79, "Station 3.Station Slide.Index"=w78) -> (w82:T1)
    }
    frame 4 {
      n33 = case shown="True" w109 {
        tunnel: ["" ("State(s) in Front (\"\")") "Door Ops 4" ("State(s) in Front (\"\")")] -> w105
        frame False {
        }
        frame True {
        }
      }
      n34 = case shown="True" w107 {
        tunnel: ["" w121] -> w113
        tunnel: w110 -> [_ w122]
        frame False {
        }
        frame True {
          n35 = Unbundle By Name(w122) -> ("Station 4.Station Cab.Status"=w121:string)
        }
      }
      n36 = case shown="True" w106 {
        tunnel: ["" w118] -> w112
        tunnel: w110 -> [_ w119]
        frame False {
        }
        frame True {
          n37 = Unbundle By Name(w119) -> ("Station 4.Station Slide.Status"=w118:string)
        }
      }
      n38 = case shown="True" w108 {
        tunnel: ["" w124] -> w114
        tunnel: w110 -> [_ w125]
        frame False {
        }
        frame True {
          n39 = Unbundle By Name(w125) -> ("Station 4.Station Freezer.Status"=w124:string)
        }
      }
      n40 = Bundle By Name(cluster=w110, "Station 4.Station Freezer.Status"=w114, "Station 4.Station Cab.Status"=w113, "Station 4.Station Slide.Status"=w112, "Station 4.Station Freezer.Index"=w104, "Station 4.Station Cab.Index"=w103, "Station 4.Station Slide.Index"=w102) -> (w111:T1)
    }
    frame 5 {
      n41 = case shown="True" w132 {
        tunnel: ["" w145] -> w137
        tunnel: w134 -> [_ w146]
        frame False {
        }
        frame True {
          n42 = Unbundle By Name(w146) -> ("Station 5.Station Cab.Status"=w145:string)
        }
      }
      n43 = case shown="True" w133 {
        tunnel: ["" w142] -> w136
        tunnel: w134 -> [_ w143]
        frame False {
        }
        frame True {
          n44 = Unbundle By Name(w143) -> ("Station 5.Station Slide.Status"=w142:string)
        }
      }
      n45 = case shown="False" w130 {
        tunnel: ["" ("State(s) in Front (\"\")") "Door Ops 5" ("State(s) in Front (\"\")")] -> w129
        frame False {
        }
        frame True {
        }
      }
      n46 = case shown="True" w131 {
        tunnel: ["" w148] -> w138
        tunnel: w134 -> [_ w149]
        frame False {
        }
        frame True {
          n47 = Unbundle By Name(w149) -> ("Station 5.Station Freezer.Status"=w148:string)
        }
      }
      n48 = Bundle By Name(cluster=w134, "Station 5.Station Freezer.Status"=w138, "Station 5.Station Cab.Status"=w137, "Station 5.Station Slide.Status"=w136, "Station 5.Station Freezer.Index"=w128, "Station 5.Station Cab.Index"=w127, "Station 5.Station Slide.Index"=w126) -> (w135:T1)
    }
    frame 6 {
      n49 = case shown="True" w153 {
        tunnel: ["" ("State(s) in Front (\"\")") "Door Ops 6" ("State(s) in Front (\"\")")] -> w154
        frame False {
        }
        frame True {
        }
      }
      n50 = case shown="True" w155 {
        tunnel: ["" w172] -> w162
        tunnel: w158 -> [_ w173]
        frame False {
        }
        frame True {
          n51 = Unbundle By Name(w173) -> ("Station 6.Station Freezer.Status"=w172:string)
        }
      }
      n52 = case shown="True" w156 {
        tunnel: ["" w169] -> w161
        tunnel: w158 -> [_ w170]
        frame False {
        }
        frame True {
          n53 = Unbundle By Name(w170) -> ("Station 6.Station Cab.Status"=w169:string)
        }
      }
      n54 = case shown="True" w157 {
        tunnel: ["" w166] -> w160
        tunnel: w158 -> [_ w167]
        frame False {
        }
        frame True {
          n55 = Unbundle By Name(w167) -> ("Station 6.Station Slide.Status"=w166:string)
        }
      }
      n56 = Bundle By Name(cluster=w158, "Station 6.Station Freezer.Status"=w162, "Station 6.Station Cab.Status"=w161, "Station 6.Station Slide.Status"=w160, "Station 6.Station Freezer.Index"=w152, "Station 6.Station Cab.Index"=w151, "Station 6.Station Slide.Index"=w150) -> (w159:T1)
    }
    frame 7 {
      n57 = case shown="True" w177 {
        tunnel: ["" w196] -> w184
        tunnel: w183 -> [_ w197]
        frame False {
        }
        frame True {
          n58 = Unbundle By Name(w197) -> ("Station 7.Station Freezer.Status"=w196:string)
        }
      }
      n59 = case shown="True" w178 {
        tunnel: ["" w193] -> w185
        tunnel: w183 -> [_ w194]
        frame False {
        }
        frame True {
          n60 = Unbundle By Name(w194) -> ("Station 7.Station Cab.Status"=w193:string)
        }
      }
      n61 = case shown="True" w179 {
        tunnel: ["" w190] -> w186
        tunnel: w183 -> [_ w191]
        frame False {
        }
        frame True {
          n62 = Unbundle By Name(w191) -> ("Station 7.Station Slide.Status"=w190:string)
        }
      }
      n63 = case shown="True" w181 {
        tunnel: ["" ("State(s) in Front (\"\")") "Door Ops 7" ("State(s) in Front (\"\")")] -> w180
        frame False {
        }
        frame True {
        }
      }
      n64 = Bundle By Name(cluster=w183, "Station 7.Station Freezer.Status"=w184, "Station 7.Station Cab.Status"=w185, "Station 7.Station Slide.Status"=w186, "Station 7.Station Freezer.Index"=w176, "Station 7.Station Cab.Index"=w175, "Station 7.Station Slide.Index"=w174) -> (w182:T1)
    }
    frame 8 {
      n65 = case shown="True" w202 {
        tunnel: ["" w217] -> w209
        tunnel: w207 -> [_ w218]
        frame False {
        }
        frame True {
          n66 = Unbundle By Name(w218) -> ("Station 8.Station Cab.Status"=w217:string)
        }
      }
      n67 = case shown="True" w203 {
        tunnel: ["" w214] -> w208
        tunnel: w207 -> [_ w215]
        frame False {
        }
        frame True {
          n68 = Unbundle By Name(w215) -> ("Station 8.Station Slide.Status"=w214:string)
        }
      }
      n69 = case shown="True" w204 {
        tunnel: ["" ("State(s) in Front (\"\")") "Door Ops 8" ("State(s) in Front (\"\")")] -> w205
        frame False {
        }
        frame True {
        }
      }
      n70 = case shown="True" w201 {
        tunnel: ["" w220] -> w210
        tunnel: w207 -> [_ w221]
        frame False {
        }
        frame True {
          n71 = Unbundle By Name(w221) -> ("Station 8.Station Freezer.Status"=w220:string)
        }
      }
      n72 = Bundle By Name(cluster=w207, "Station 8.Station Freezer.Status"=w210, "Station 8.Station Cab.Status"=w209, "Station 8.Station Slide.Status"=w208, "Station 8.Station Freezer.Index"=w200, "Station 8.Station Cab.Index"=w199, "Station 8.Station Slide.Index"=w198) -> (w206:T1)
    }
  }
  "States" <- w18
  n73 = Equal?(x="Freezer Index", y=-1) -> (x = y?=w9:bool)
  n74 = Equal?(x="Cab Index", y=-1) -> (x = y?=w8:bool)
  n75 = Equal?(x="Slide Index", y=-1) -> (x = y?=w7:bool)
  n76 = Compound Arithmetic op=AND(w9, w8, w7) -> (w6:bool)
  n77 = call "RTS End Test Logging.vi"("All Door Opener Ctrl Input"=w5, "RTS Config Setup Input"="RTS Config Setup Input", "Times Up?"=w6, "Error In"="Error In", "Station #"="Station #") -> ("All Door Opener Ctrl Output"=→"All Door Opener Ctrl Out":T1, "RTS Config Setup Output"=→"RTS Config Setup Output":T7, "Error Out"=→"Error Out":errorcluster)  [unwired: 8 in]
